vi "Redirect.vi"(7 "LabVIEW Web Service Request":refnum<class "Web Request.lvclass">, 11 "package":string) -> ()   [LabVIEW 2016]
uses:
  <vilib>/wsapi/Web Request.lvclass
  <vilib>/wsapi/class/subVIs/Write Single Session Variable.vi
  Libraries/WSsupport/WSsupport.lvlib
  Libraries/ServerErrors/ServerErrors.lvlib
panel:
  # "Use the Web Service Request input terminal to call the VIs on the Web Services palette. Do not remove it from the connector pane unless you don't need access to the palette."
  # "Each additional control wired to the connector pane will be available as an input in the URL. To include an indicator in terminal-mode output (the default setting), it must also be wired to the connector pane."
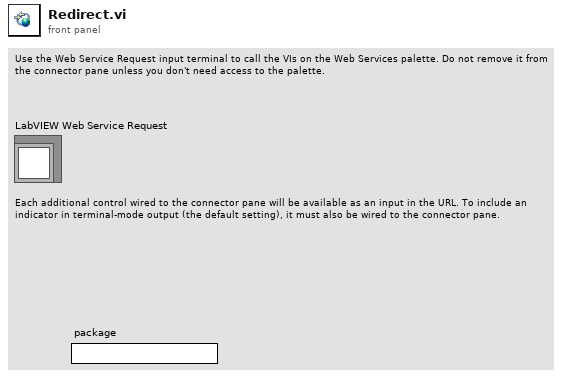
[diagram p1: front panel]
types:
  T1 = typedef "ServerErrors.lvlib/Error Message--cluster.ctl" = cluster{"HTTP Code":i32, "JSON Response":cluster{"error":string, "reason":string}}
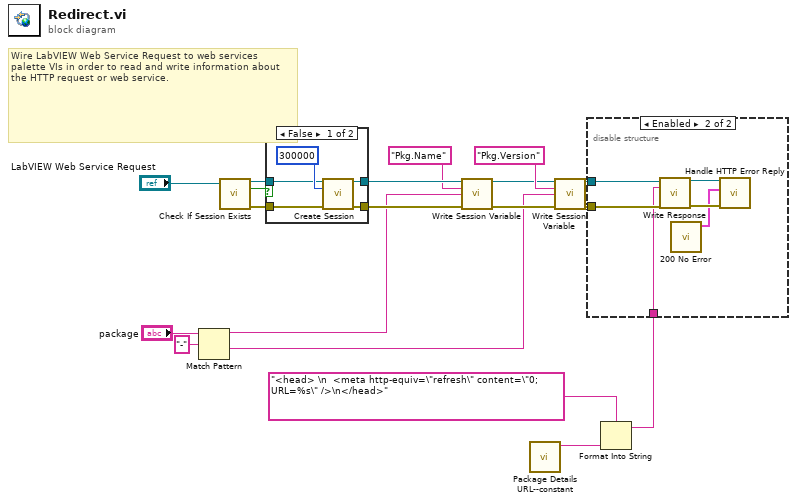
[diagram p0: block diagram]
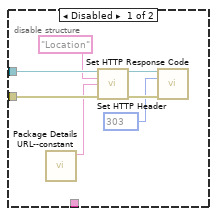
[diagram p2: hidden frame]
diagram:
  # "Wire LabVIEW Web Service Request to web services palette VIs in order to read and write information about the HTTP request or web service."
  n1 = Match Pattern(string="package", regular expression="-") -> (before substring=w7:string, after substring=w6:string)  [unwired: 1 in, 2 out]
  n2 = call <vilib>:"Check If Session Exists.vi"("LabVIEW Web Service Request"="LabVIEW Web Service Request") -> ("LabVIEW Web Service Request out"=w12:refnum<class "Web Request.lvclass">, "session exists?"=w11:bool, "error out"=w13:errorcluster)  [unwired: 12 in]
  n3 = case shown="False" w11 {
    tunnel: [w23 w26] -> w19
    tunnel: [w22 w25] -> w18
    tunnel: w13 -> [w21 w25]
    tunnel: w12 -> [w20 w26]
    frame False {
      n4 = call <vilib>:"Create Session.vi"("LabVIEW Web Service Request"=w20, "timeout (60000 msec)"=u32 300000, "error in (no error)"=w21) -> ("LabVIEW Web Service Request out"=w23:refnum<class "Web Request.lvclass">, "error out"=w22:errorcluster)  [unwired: 10 in, 1 out]
    }
    frame True {
    }
  }
  n5 = call-poly <vilib>:"Write Session Variable.vi"("LabVIEW Web Service Request"=w19, "key"="Pkg.Name", "value"=w7, "error in (no error)"=w18) -> ("LabVIEW Web Service Request out"=w15:refnum<class "Web Request.lvclass">, "error out"=w14:errorcluster)  [unwired: 8 in, 2 out]
  n6 = call "Package Details URL--constant.vi"() -> ("Package Details URL"=w2:string)  [unwired: 11 in]
  n7 = call-poly <vilib>:"Write Session Variable.vi"("LabVIEW Web Service Request"=w15, "key"="Pkg.Version", "value"=w6, "error in (no error)"=w14) -> ("LabVIEW Web Service Request out"=w5:refnum<class "Web Request.lvclass">, "error out"=w4:errorcluster)  [unwired: 8 in, 2 out]
  n8 = Format Into String(format string="<head> \n  <meta http-equiv=\"refresh\" content=\"0; URL=%s\" />\n</head>", w2) -> (resulting string=w1:string)  [unwired: 2 in, 1 out]
  n9 = disable-structure shown="Enabled" {
    disable-tunnel: w5 -> [w33 w39]
    disable-tunnel: w4 -> [w32 w38]
    disable-tunnel: w1 -> [_ w37]
    frame Disabled {
      w27 = 303 items=["100"=100, "101"=101, "200"=200, "201"=201, "202"=202, "203"=203, "204"=204, "205"=205, "206"=206, "300"=300, "301"=301, "302"=302, "303"=303, "304"=304, "305"=305, "306"=306, "307"=307, "400"=400, "401"=401, "402"=402, "403"=403, "404"=404, "405"=405, "406"=406, "407"=407, "408"=408, "409"=409, "410"=410, "411"=411, "412"=412, "413"=413, "414"=414, "415"=415, "416"=416, "417"=417, "500"=500, "501"=501, "502"=502, "503"=503, "504"=504, "505"=505] ("response code (307)")
      n10 = call "Package Details URL--constant.vi"() -> ("Package Details URL"=w31:string)  [unwired: 11 in]
      n11 = call <vilib>:"Set HTTP Header.vi"("LabVIEW Web Service Request"=w33, "header"="Location", "header value"=w31, "error in (no error)"=w32) -> ("LabVIEW Web Service Request out"=w29:refnum<class "Web Request.lvclass">, "error out"=w28:errorcluster)  [unwired: 10 in]
      n12 = call <vilib>:"Set HTTP Response Code.vi"("LabVIEW Web Service Request"=w29, "response code (200)"=w27, "error in (no error)"=w28) -> ()  [unwired: 11 in, 2 out]
    }
    frame Enabled {
      n13 = call <vilib>:"Write Response.vi"("LabVIEW Web Service Request"=w39, "response string"=w37, "error in (no error)"=w38) -> ("LabVIEW Web Service Request out"=w36:refnum<class "Web Request.lvclass">, "error out"=w35:errorcluster)  [unwired: 11 in]
      n14 = call "200 No Error.vi"() -> ("no error"=w34:T1)  [unwired: 11 in]
      n15 = call "Handle HTTP Error Reply.vi"("error in (no error)"=w35, "HTTP Status Code"=w34, "Web Request in"=w36) -> ()  [unwired: 8 in, 1 out]
    }
  }
